vi "写入input.vi"(8 "error in (no error)":errorcluster caption="错误输入（无错误）", 10 "input":T1, 11 "WebDAV client输入":refnum<class "WebDAV client.lvclass">) -> (0 "error out":errorcluster caption="错误输出", 3 "WebDAV client输出":refnum<class "WebDAV client.lvclass">)   [LabVIEW 2016, in "数据传输系统-03.lvlib" / "update.lvlib" / "WebDAV client.lvclass"]
uses:
  WebDAV client.lvclass
  WebDAV client.lvclass/WebDAV client.ctl
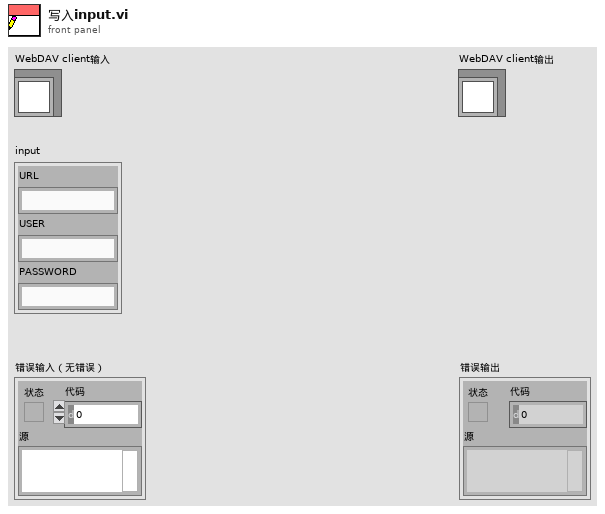
[diagram p1: front panel]
types:
  T1 = cluster{"URL":string, "USER":string, "PASSWORD":string}
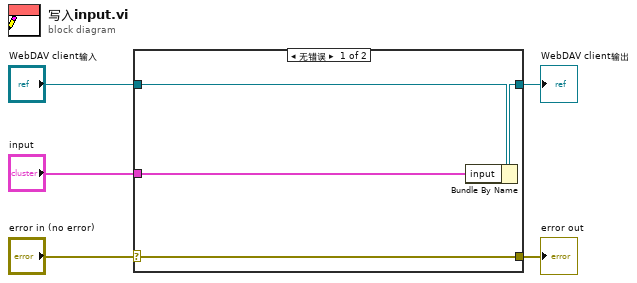
[diagram p0: block diagram]
diagram:
  n1 = case shown="无错误" "error in (no error)" {
    selector: "error in (no error)" -> [w9 w10]
    tunnel: [w9 w10] -> w4
    tunnel: [w7 w11] -> w2
    tunnel: "WebDAV client输入" -> [w8 w11]
    tunnel: "input" -> [w6 _]
    frame No Error {
      n2 = Bundle By Name(cluster=w8, "input"=w6) -> (w7:refnum<class "WebDAV client.lvclass">)
    }
    frame Error {
    }
  }
  "error out" <- w4
  "WebDAV client输出" <- w2
